vi "raw_torque_to_mA_and_kN.vi"(8 "Max Motor Torque Nm":dbl, 9 "Max Motor Current mA":dbl, 11 "Torque % raw":i32) -> (0 "Motor Torque Nm":dbl, 1 "Motor Current mA":dbl, 3 "Torque %":dbl)   [LabVIEW 2021]
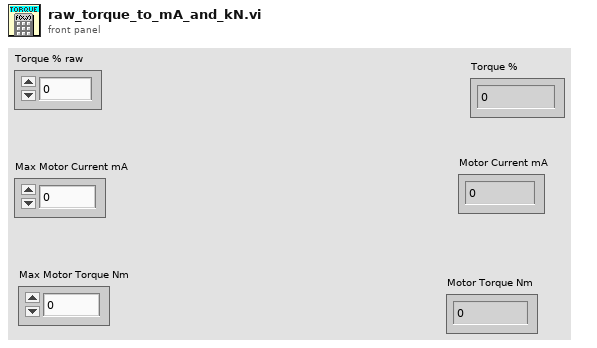
[diagram p1: front panel]
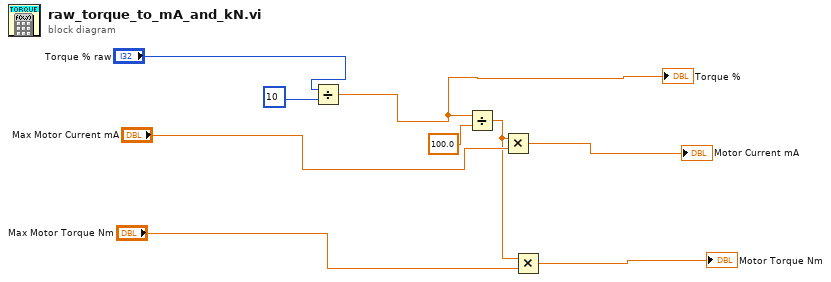
[diagram p0: block diagram]
diagram:
  n1 = Divide(x="Torque % raw", y=10) -> (x/y=w1:dbl)
  "Torque %" <- w1
  n2 = Divide(x=w1, y=100.0) -> (x/y=w3:dbl)
  n3 = Multiply(x=w3, y="Max Motor Current mA") -> (x*y=→"Motor Current mA":dbl)
  n4 = Multiply(x=w3, y="Max Motor Torque Nm") -> (x*y=→"Motor Torque Nm":dbl)
